vi "MQTT_Simple_Connect_and_Subscribe.vi"() -> ()   [LabVIEW 2024, in "MQTT_Functions.lvlib"]
doc: "A basic client example that connects to a server, subscribes to a variety of topics and receives responses for the topics. \n\n© 2015 - daq.io, LLC - Peter Adelhardt"
uses:
  MQTT_Functions.lvlib
  Controls/Connect_Flags.ctl
  Controls/QoS.ctl
  Controls/Connection_Return_Codes.ctl
  Controls/MessageType.ctl
  Controls/DUP_Flag.ctl
  Controls/Retain_Flag.ctl
panel:
  out "Messages":T2(array[cluster])
  in  "Stop Reading":bool
  in  "MQTT Broker":cluster{"address (IP)":string, "port":u16}={"address (IP)"="10.20.1.20", "port"=1883}
  in  "Subscription Info Array":cluster{"Topic":string, "QoS":T3}[](array[cluster])=[{"Topic"="testtopic/LVMQTT", "QoS"=enum."At most once"}]
  out "Granted QoS Levels":T3[](array[typedef])
  out "Connection Status":T4=enum."Connection refused: Server unavailable"
  in  "Connect Flags":T5
  in  "Client ID":string="LVSubscribeClient"
  out "error out":errorcluster
  in  "error in (no error)":errorcluster
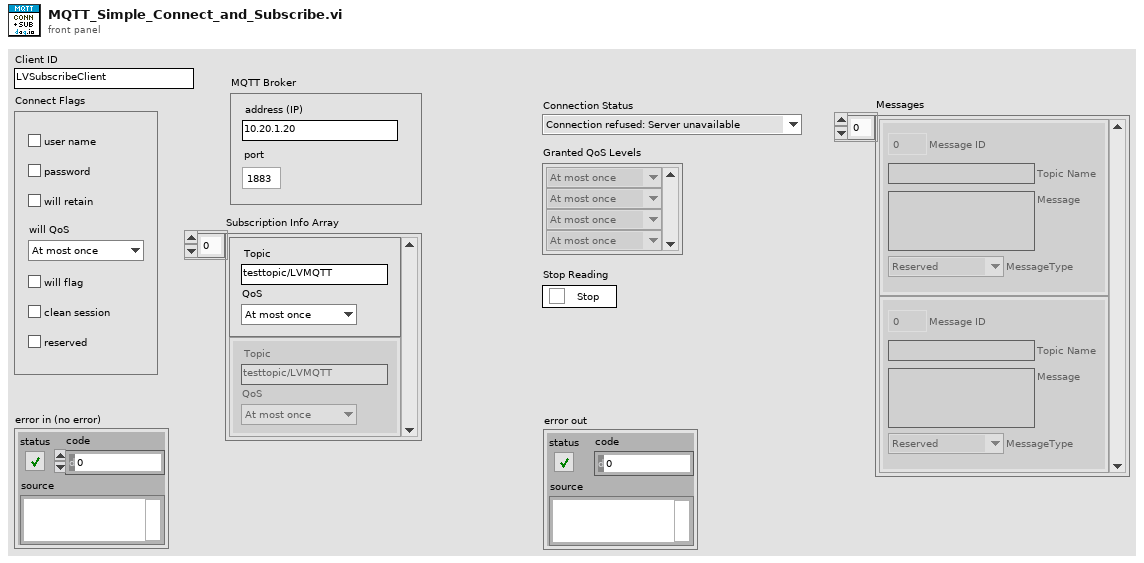
[diagram p1: front panel]
types:
  T1 = typedef "MQTT_Functions.lvlib/MessageType.ctl" = enum32{"Reserved", "CONNECT", "CONNACK", "PUBLISH", "PUBACK", "PUBREC", "PUBREL", "PUBCOMP", "SUBSCRIBE", "SUBACK", "UNSUBSCRIBE", "UNSUBACK", "PINGREQ", "PINGRESP", "DISCONNECT", "Reserved2"}
  T2 = cluster{"Message ID":u16, "Topic Name":string, "Message ":string, "MessageType":T1}[]
  T3 = typedef "MQTT_Functions.lvlib/QoS.ctl" = enum8{"At most once", "At least once", "Exactly once", "Reserved"}
  T4 = typedef "MQTT_Functions.lvlib/Connection_Return_Codes.ctl" = enum16{"Connection accepted", "Connection refused: unacceptable protocol version", "Connection refused: identifier rejected", "Connection refused: Server unavailable", "Connection refused: bad user name or password", "Connection refused: not authorized"}
  T5 = typedef "MQTT_Functions.lvlib/Connect_Flags.ctl" = cluster{"user name":bool, "password":bool, "will retain":bool, "will flag":bool, "clean session":bool, "reserved":bool, "will QoS":T3}
  T6 = cluster{"Message ID":u16, "Topic Name":string, "Message":string, "MessageType":T1}[]
  T7 = typedef "MQTT_Functions.lvlib/DUP_Flag.ctl" = bool
  T8 = typedef "MQTT_Functions.lvlib/Retain_Flag.ctl" = bool
  T9 = cluster{"QoS":T3, "DUP":T7, "Retain":T8, "Keep Alive (sec)":u16}
  T10 = cluster{"Message ID":u16, "Topic Name":string, "Message":string, "MessageType":T1}
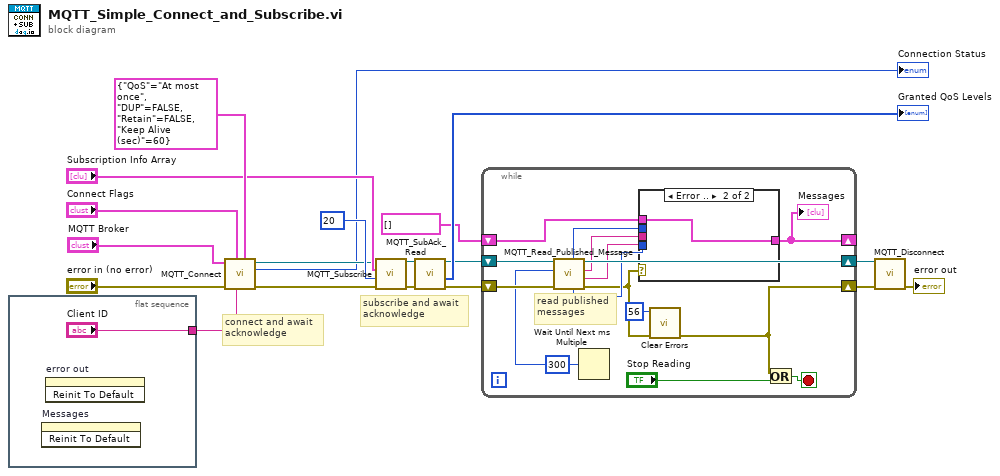
[diagram p0: block diagram]
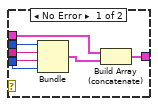
[diagram p2: hidden frame]
diagram:
  # "connect and await\nacknowledge"
  # "subscribe and await\nacknowledge"
  n1 = flat-sequence {
    tunnel: ["Client ID"] -> w19
    frame #0 {
      n2 = invoke on="Messages" class="Arr (strict)" method="Reinit To Default"() -> ()  [unwired: 3 in, 3 out]
      n3 = invoke on="error out" class="Clust (strict)" method="Reinit To Default"() -> ()  [unwired: 3 in, 3 out]
    }
  }
  n4 = call "MQTT_Connect.vi"("Connect Meta"=T9 {"QoS"=enum."At most once", "DUP"=FALSE, "Retain"=FALSE, "Keep Alive (sec)"=60}, "Client ID"=w19, "Connect Flags"="Connect Flags", "error in (no error)"="error in (no error)", "MQTT Broker"="MQTT Broker") -> ("error out"=w1:errorcluster, "Connection Status"=→"Connection Status":T4, "connection ID out"=w3:refnum<k5>)  [unwired: 4 in]
  n5 = call "MQTT_Subscribe.vi"("error in (no error)"=w1, "Message ID"=u16 20, "Subscription Info Array"="Subscription Info Array", "connection ID"=w3) -> ("error out"=w12:errorcluster, "connection ID out"=w13:refnum<k5>)  [unwired: 6 in]
  n6 = call "MQTT_SubAck_Read.vi"("error in (no error)"=w12, "connection ID"=w13) -> ("error out"=w10:errorcluster, "Granted QoS Levels"=→"Granted QoS Levels":T3[], "connection ID out"=w9:refnum<k5>)  [unwired: 7 in]
  n7 = while {
    shift-right: [w25] -> _
    shift-left: T6 [] ("Array") -> [w26]
    shift-right: [w23] -> w7
    shift-left: w10 -> [w35]
    shift-right: [w33] -> w8
    shift-left: w9 -> [w34]
    stop <- w28 stop-if-true
    w21 = u32 300 ("millisecond multiple")
    # "read published\nmessages"
    n8 = call "MQTT_Read_Published_Message.vi"("error in (no error)"=w35, "timeout ms (25000)"=w21, "connection ID"=w34) -> ("error out"=w22:errorcluster, "Message"=w30:string, "Topic Name"=w31:string, "connection ID out"=w33:refnum<k5>, "MessageType"=w29:T1, "Message ID"=w32:u16)  [unwired: 3 in]
    n9 = Wait Until Next ms Multiple(millisecond multiple=w21) -> ()  [unwired: 1 out]
    n10 = case shown="Error .." w22 {
      tunnel: w32 -> [w42 _]
      tunnel: w31 -> [w41 _]
      tunnel: w30 -> [w40 _]
      tunnel: w29 -> [w39 _]
      tunnel: w26 -> [w38 w43]
      tunnel: [w36 w43] -> w25
      frame No Error {
        n11 = Bundle("Message ID"=w42, "Topic Name"=w41, "Message"=w40, "MessageType"=w39) -> (w37:T10)  [unwired: 1 in]
        n12 = Build Array (concatenate)(w38, w37) -> (w36:T6)
      }
      frame Error {
      }
    }
    "Messages" <- w25
    n13 = call <vilib>:"Clear Errors.vi"("error in (no error)"=w22, "specific error code to clear (0: all)"=56) -> ("error out"=w23:errorcluster)  [unwired: 4 in, 1 out]
    n14 = Or(x=w23, y="Stop Reading") -> (x .or. y?=w28:bool)
  }
  n15 = call "MQTT_Disconnect.vi"("error in (no error)"=w7, "connection ID"=w8) -> ("error out"=→"error out":errorcluster)  [unwired: 9 in]
